vi "Handle Error.vi"(8 "error in (no error)":errorcluster, 9 "Error":errorcluster, 10 "Error Level":T1, 11 "ATM Controller in":refnum<class "ATM Controller.lvclass">) -> (0 "error out":errorcluster, 3 "ATM Controller out":refnum<class "ATM Controller.lvclass">)   [LabVIEW 2019, in "ATM Controller.lvlib" / "ATM Controller.lvclass"]
uses:
  ATM Controller.lvclass
  Error Level.ctl
  Error Data.ctl
  ATM Controller Messages/Set State Msg/Set State Msg.lvclass
  <vilib>/ActorFramework/Actor/Actor.lvclass
  State -Enum.ctl
  C:/Program Files (x86)/National Instruments/LabVIEW 2019/vi.lib/ActorFramework/Actor/Actor.lvclass
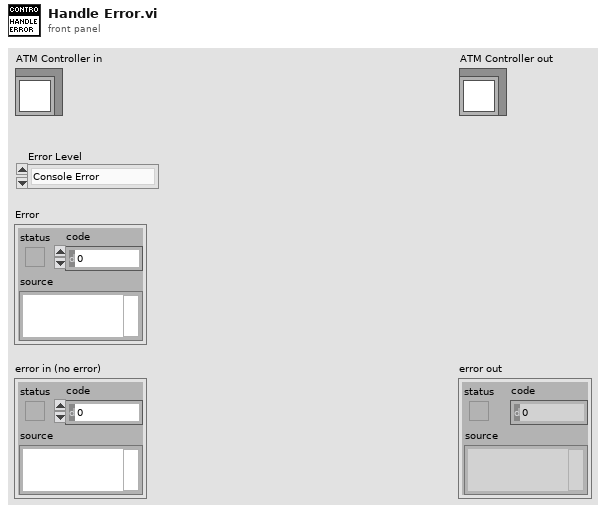
[diagram p1: front panel]
types:
  T1 = typedef "ATM Controller.lvlib/ATM Controller.lvclass/Error Level.ctl" = enum16{"Console Error", "Sensor Interface IO Error", "Process Step Error"}
  T2 = typedef "ATM Controller.lvlib/ATM Controller.lvclass/Error Data.ctl" = cluster{"Description":string, "Error Level":T1, "Time Stamp":timestamp}
  T3 = typedef "ATM Controller.lvlib/ATM Controller.lvclass/State -Enum.ctl" = enum16{"Initial", "Idle", "Login", "Balance Inquiry", "Deposit", "Withdrawal", "Fast Cash", "Terminate", "Inactivity Timeout"}
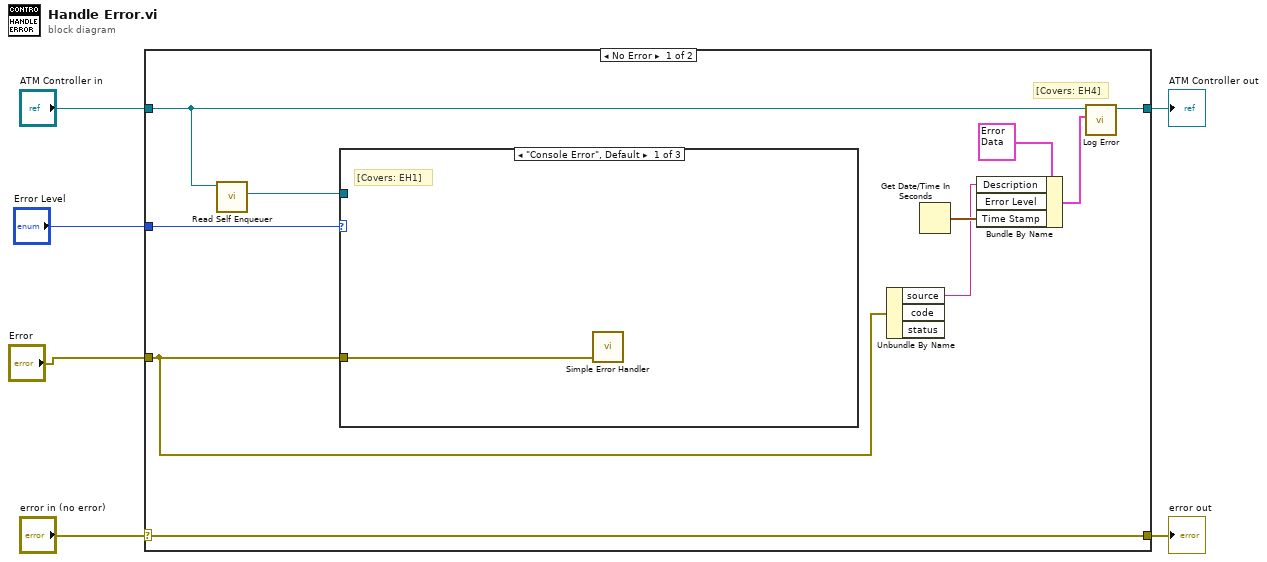
[diagram p0: block diagram]
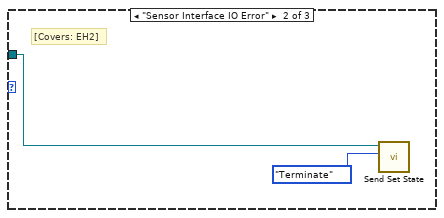
[diagram p2: hidden frame]
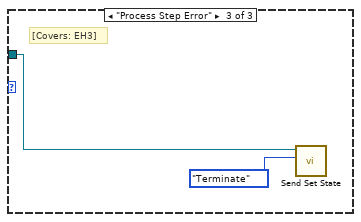
[diagram p3: hidden frame]
diagram:
  n1 = case shown="No Error" "error in (no error)" {
    selector: "error in (no error)" -> [w16 w23]
    tunnel: [w16 w23] -> w5
    tunnel: [w15 w22] -> w3
    tunnel: "ATM Controller in" -> [w10 w22]
    tunnel: "Error Level" -> [w11 _]
    tunnel: "Error" -> [w7 _]
    frame No Error {
      # "[Covers: EH4]"
      n2 = call <vilib>:"Read Self Enqueuer.vi"("Actor"=w10) -> ("Self Enqueuer"=w9:refnum<class "Message Enqueuer.lvclass">)  [unwired: 10 in]
      n3 = case shown="\"Console Error\", Default" w11 {
        tunnel: w9 -> [_ w19 w20]
        tunnel: w7 -> [w17 _ _]
        frame "Console Error", Default {
          # "[Covers: EH1]"
          n4 = call <vilib>:"Simple Error Handler.vi"("error in (no error)"=w17) -> ()  [unwired: 4 in, 5 out]
        }
        frame "Sensor Interface IO Error" {
          # "[Covers: EH2]"
          n5 = call "Send Set State.vi"("State"=State_-Enum."Terminate", "Message Enqueuer"=w19) -> ()  [unwired: 8 in, 2 out]
        }
        frame "Process Step Error" {
          # "[Covers: EH3]"
          n6 = call "Send Set State.vi"("State"=State_-Enum."Terminate", "Message Enqueuer"=w20) -> ()  [unwired: 8 in, 2 out]
        }
      }
      n7 = Unbundle By Name(w7) -> ("source"=w8:string)  [unwired: 2 out]
      n8 = Get Date/Time In Seconds() -> (seconds since 1Jan1904=w12:timestamp)
      n9 = Bundle By Name(cluster=T2 {"Description"="", "Error Level"=enum."Console Error", "Time Stamp"=timestamp(0 s since 1904-01-01)} ("Error Data"), "Description"=w8, "Time Stamp"=w12) -> (w13:T2)  [unwired: 1 in]
      n10 = call "Log Error.vi"("Error Data"=w13, "ATM Controller in"=w10) -> ("ATM Controller out"=w15:refnum<class "ATM Controller.lvclass">)  [unwired: 8 in, 1 out]
    }
    frame Error {
    }
  }
  "error out" <- w5
  "ATM Controller out" <- w3
